vi "Connection Put Data.vi"(8 "error in (no error)":errorcluster, 9 "Path in":string, 10 "Data":refnum<data-value>, 11 "Connection DVR in":refnum<data-value>) -> (0 "error out":errorcluster, 3 "Connection DVR out":refnum<data-value>)   [LabVIEW 2015, in "MDSplus.lvlib"]
uses:
  <vilib>/MDSplus/Library/MDSplus.lvlib
  <vilib>/MDSplus/Classes/Data_Class/Data.lvclass
  <vilib>/MDSplus/Classes/Connection_Class/Connection.lvclass
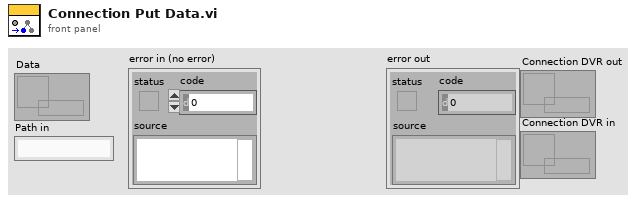
[diagram p1: front panel]
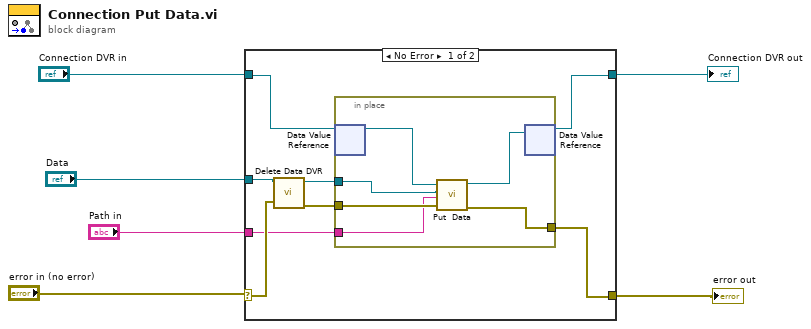
[diagram p0: block diagram]
diagram:
  n1 = case shown="No Error" "error in (no error)" {
    selector: "error in (no error)" -> [w9 w21]
    tunnel: "Connection DVR in" -> [w14 w22]
    tunnel: [w13 w22] -> w4
    tunnel: [w12 w21] -> w3
    tunnel: "Data" -> [w11 _]
    tunnel: "Path in" -> [w7 _]
    frame No Error {
      n2 = call <vilib>:"Delete Data DVR.vi"("error in (no error)"=w9, "Data DVR in"=w11) -> ("error out"=w8:errorcluster, "Data out"=w10:refnum<class "Data.lvclass">)  [unwired: 8 in]
      n3 = in-place {
        in-place-border: [w18] -> w12
        in-place-border: w10 -> [w17]
        in-place-border: w8 -> [w16]
        in-place-border: w7 -> [w15]
        n4 = in-place-dvr #1(w14) -> (w20:refnum<class "Connection.lvclass">)  [unwired: 1 out]
        n5 = call <vilib>:"Put  Data.vi"("error in (no error)"=w16, "Path in"=w15, "Data"=w17, "Connection in"=w20) -> ("error out"=w18:errorcluster, "Connection out"=w19:refnum<class "Connection.lvclass">)  [unwired: 6 in]
        n6 = in-place-dvr #1(w19) -> (w13:refnum<data-value>)  [unwired: 1 out]
      }
    }
    frame Error {
    }
  }
  "error out" <- w3
  "Connection DVR out" <- w4
